vi "Create_Simple_Var.vi"(4 "Value":T1) -> (1 "Var":refnum<class "Var_I8.lvclass">)   [LabVIEW 2021, in "Var_I8.lvclass"]
uses:
  Var_I8.lvclass
  Type.ctl
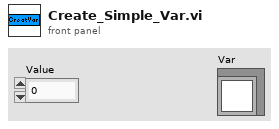
[diagram p1: front panel]
types:
  T1 = typedef "Var_I8.lvclass/Type.ctl" = i8
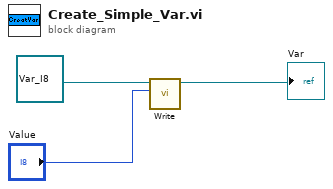
[diagram p0: block diagram]
diagram:
  n1 = call-dynamic "Write.vi"("Value"="Value", "Double Float.lvclass_340760 in"=refnum<class "Var_I8.lvclass"> refnum ("Constants.lvlib:Numeric.lvclass")) -> ("Double Float.lvclass_340760 out"=→"Var":refnum<class "Var_I8.lvclass">)  [unwired: 8 in, 1 out]
